vi "Reset Eload.vi"(8 "error in":errorcluster, 11 "3300 in":refnum<class "3300.lvclass">) -> (0 "error out":errorcluster, 3 "3300 out":refnum<class "3300.lvclass">)   [LabVIEW 2019, in "3300.lvlib" / "3300.lvclass"]
uses:
  Library/3300.lvclass
  builds/Instruments/Electronic Load.lvlibp/Library/Electronic Load.lvclass
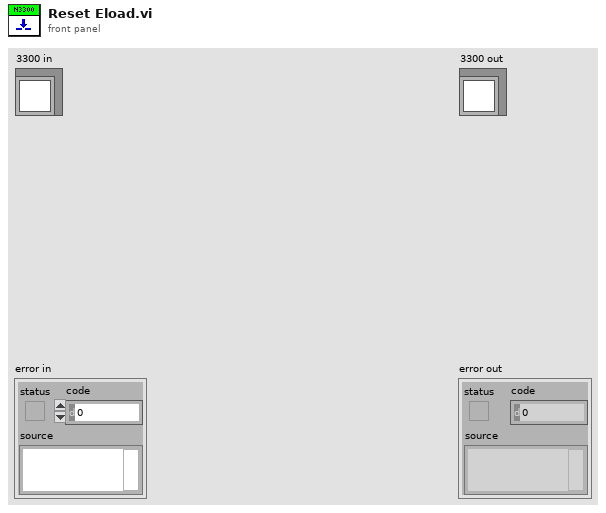
[diagram p1: front panel]
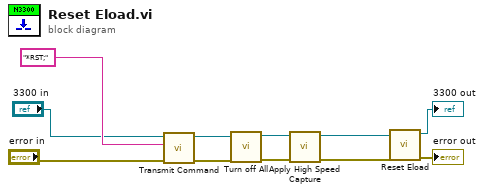
[diagram p0: block diagram]
diagram:
  n1 = call "Transmit Command.vi"("error in"="error in", "Command"="*RST;", "3300 in"="3300 in") -> ("error out"=w7:errorcluster, "3300 out"=w8:refnum<class "3300.lvclass">)  [unwired: 7 in]
  n2 = call-dynamic "Turn off All.vi"("error in"=w7, "3300 in"=w8) -> ("error out"=w5:errorcluster, "3300 out"=w6:refnum<class "3300.lvclass">)  [unwired: 8 in]
  n3 = call "Apply High Speed Capture.vi"("error in"=w5, "3300 in"=w6) -> ("error out"=w2:errorcluster, "3300 out"=w3:refnum<class "3300.lvclass">)  [unwired: 8 in]
  n4 = call-parent "Reset Eload.vi"("error in"=w2, "Electronic Load in"=w3) -> ("error out"=→"error out":errorcluster, "Electronic Load out"=→"3300 out":refnum<class "3300.lvclass">)  [unwired: 8 in]
